vi "Trial_status_text.vi"(10 "Protocol cluster":T1, 11 "Trial sequence":cluster{"Sequence name":string, "Active":bool}[](array[cluster])) -> (3 "Trials status text":string)   [LabVIEW 2016]
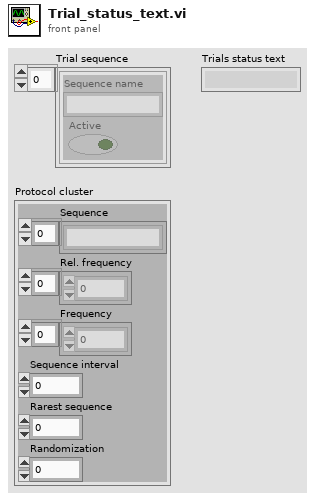
[diagram p1: front panel]
types:
  T1 = cluster{"Sequence":string[], "Rel. frequency":u32[], "Frequency":dbl[], "Sequence interval":dbl, "Rarest sequence ":dbl, "Randomization":u16}
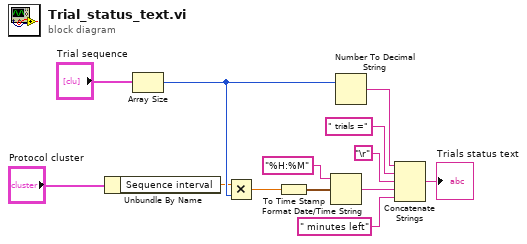
[diagram p0: block diagram]
diagram:
  n1 = Unbundle By Name("Protocol cluster") -> ("Sequence interval"=w7:dbl)
  n2 = Array Size(array="Trial sequence") -> (size(s)=w8:i32)
  n3 = Multiply(x=w7, y=w8) -> (x*y=w9:dbl)
  n4 = To Time Stamp(1:w9) -> (0:w11:timestamp)
  n5 = Format Date/Time String(time format string (%c)="%H:%M", seconds (now)=w11) -> (date/time string=w12:string)  [unwired: 1 in]
  n6 = Number To Decimal String(number=w8) -> (decimal integer string=w2:string)  [unwired: 1 in]
  n7 = Concatenate Strings(w2, " trials =" ("string"), "\r", w12, " minutes left" ("string")) -> (→"Trials status text":string)
